vi "Ballast.vi"(11 "Full System Configuration":T1={"Rack"=enum."15U; 1-Phase; 16A; 100-240V", "Middle Rail"=enum."None", "Ballast"={"Main"=0, "Small"=0, "Side"=0}, "Front Panel I/O"={"EMO Button"=FALSE, "USB 3.0"=FALSE, "Display"=FALSE, "1st USB 2.0"=FALSE, "2nd USB 2.0"=FALSE, "Ethernet 3"=FALSE, "EMO Extension (3rd Party)"=FALSE, "EMO Extension (Rack In & Out)"=FALSE, "Aux Dual C13 QAC Outlets"=FALSE, "Residual-current Circuit Breaker"=FALSE, "Serial"=FALSE, "GPIB"=FALSE}, "Rear Panel I/O"={"Rear Panel I/O Configuration"=enum."Blank Panel", "EMO Button"=FALSE, "Power, Status & Banana Ground"=FALSE, "Ethernet 2"=FALSE, "Display"=FALSE, "USB 3.0"=FALSE, "DIO"=FALSE, "GPIB"=FALSE, "Aux Dual C13 QAC Outlets"=FALSE, "Residual-current Circuit Breaker"=FALSE, "Serial"=FALSE, "SMA"=FALSE}, "Miscellaneous Options"={"Eyebolts"=FALSE, "Tower Light"=FALSE, "Top/Side Monitor Mount Kit"=FALSE, "24\" Monitor"=FALSE, "Keyboard & Mouse"=FALSE, "Secondary Ethernet Switch"=FALSE, "Extra USB Hub"=FALSE, "USB-6509"=FALSE, "Front Door"=enum."38U (Solid) IG", "Primary Ethernet Switch"=enum."Item 0", "Use Posture"=enum."Item 0"}, "Accessories"={"Screw Type"=enum."10-32", "Cage Nuts & Screws"=0.0, "Filler Panel Color"=enum."Interface Gray", "1U"=0.0, "2U"=0.0, "3U"=0.0}} {"Ballast"."Side" max=5 step=1; "Ballast"."Small" max=5 step=1; "Ballast"."Main" max=5 step=1}) -> (3 "Array":T13[](array[typedef]))   [LabVIEW 2023]
uses:
  Option Type Defs/Parts List.ctl
  Option Type Defs/Full System Configuration.ctl
  Option Type Defs/Rack.ctl
  Option Type Defs/Middle Rail.ctl
  Option Type Defs/Ballast.ctl
  Option Type Defs/Front Panel IO.ctl
  Option Type Defs/Rear Panel IO.ctl
  Option Type Defs/Rear Panel IO Configuration.ctl
  Option Type Defs/Miscellaneous Options.ctl
  Option Type Defs/Front Door.ctl
  Option Type Defs/Accessories.ctl
  Option Type Defs/Screw Types.ctl
  Option Type Defs/Filler Panel Color.ctl
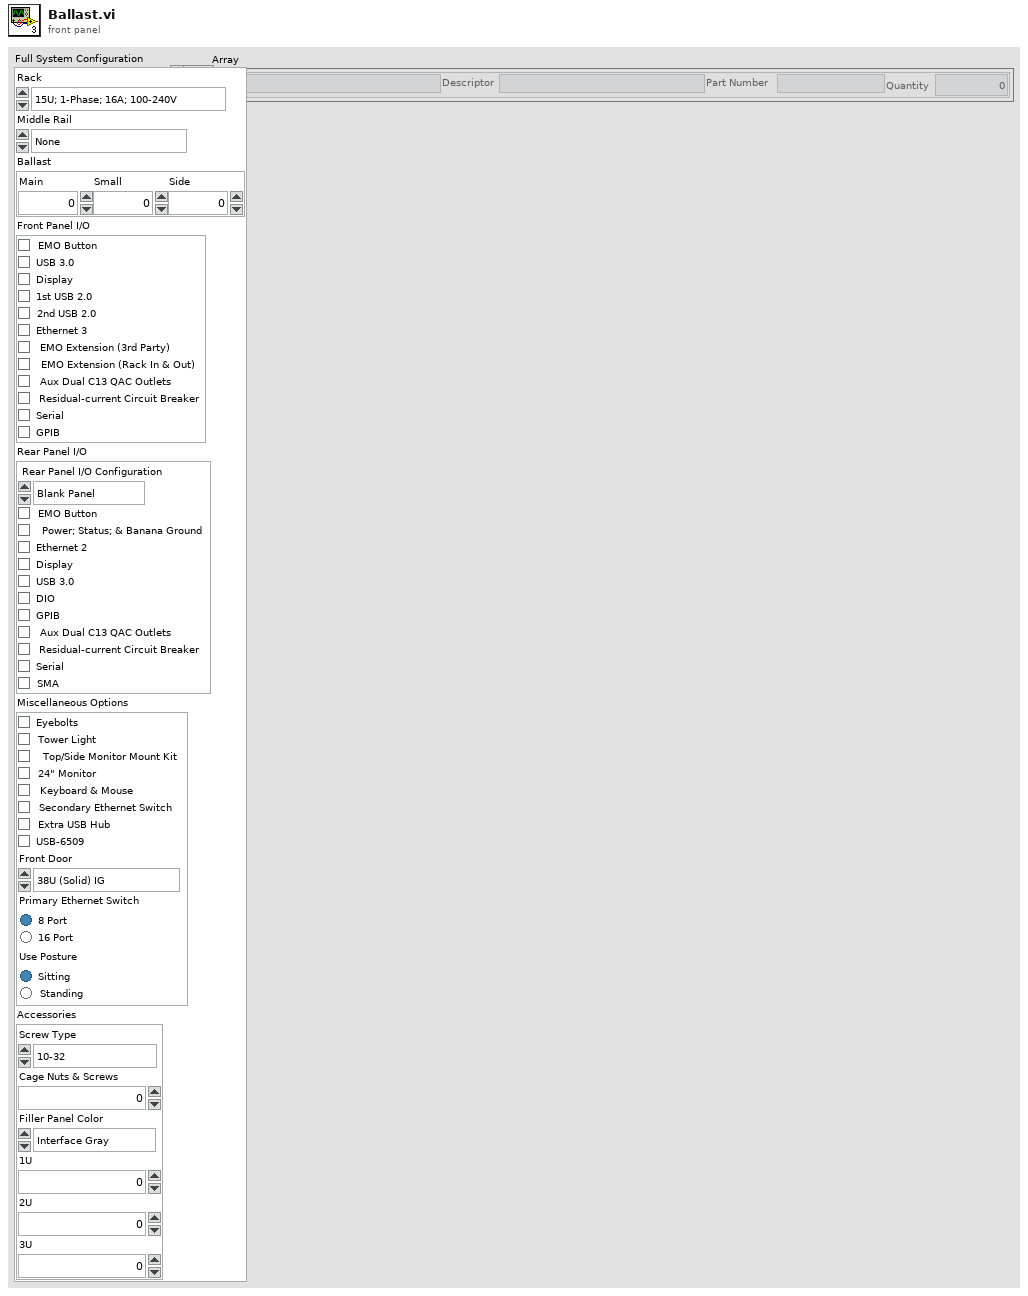
[diagram p1: front panel]
types:
  T1 = typedef "Full System Configuration.ctl" = cluster{"Rack":T2, "Middle Rail":T3, "Ballast":T4, "Front Panel I/O":T5, "Rear Panel I/O":T6, "Miscellaneous Options":T8, "Accessories":T10}
  T2 = typedef "Rack.ctl" = enum16{"15U; 1-Phase; 16A; 100-240V", "15U; 1-Phase; 24A; 100-240V", "38U; 3-Phase Delta; 50A; 200-240V", "38U; 1-Phase; 24A; 100-120V", "38U; 3-Phase Wye; 50A; 200-240V", "38U; 3-Phase Delta; 50A; 380-480V", "38U; 3-Phase Delta; 32A; 200-240V", "38U; 3-Phase Wye; 16A; 100-240V", "44U; 1-Phase; 24A; 100-240V", "44U; 3-Phase Delta; 32A; 200-240V"}
  T3 = typedef "Middle Rail.ctl" = enum16{"None", "Flip Side Rear; D=168.83mm", "Parallel Rear; D=145mm", "Flip Side Front; D=145mm", "Parallel Front; D=145mm"}
  T4 = typedef "Ballast.ctl" = cluster{"Main":u16, "Small":u16, "Side":u16}
  T5 = typedef "Front Panel IO.ctl" = cluster{"EMO Button":bool, "USB 3.0":bool, "Display":bool, "1st USB 2.0":bool, "2nd USB 2.0":bool, "Ethernet 3":bool, "EMO Extension (3rd Party)":bool, "EMO Extension (Rack In & Out)":bool, "Aux Dual C13 QAC Outlets":bool, "Residual-current Circuit Breaker":bool, "Serial":bool, "GPIB":bool}
  T6 = typedef "Rear Panel IO.ctl" = cluster{"Rear Panel I/O Configuration":T7, "EMO Button":bool, "Power, Status & Banana Ground":bool, "Ethernet 2":bool, "Display":bool, "USB 3.0":bool, "DIO":bool, "GPIB":bool, "Aux Dual C13 QAC Outlets":bool, "Residual-current Circuit Breaker":bool, "Serial":bool, "SMA":bool}
  T7 = typedef "Rear Panel IO Configuration.ctl" = enum16{"Blank Panel", "Fully Populated Panel", "Custom Panel"}
  T8 = typedef "Miscellaneous Options.ctl" = cluster{"Eyebolts":bool, "Tower Light":bool, "Top/Side Monitor Mount Kit":bool, "24\" Monitor":bool, "Keyboard & Mouse":bool, "Secondary Ethernet Switch":bool, "Extra USB Hub":bool, "USB-6509":bool, "Front Door":T9, "Primary Ethernet Switch":enum32{"Item 0", "Item 1"}, "Use Posture":enum32{"Item 0", "Item 1"}}
  T9 = typedef "Front Door.ctl" = enum16{"None", "38U (Solid) IG", "38U (Solid) EG", "38U: Top 14U (Solid) IG", "38U (Clear) IG", "44U (Solid) IG", "44U (Solid) EG"}
  T10 = typedef "Accessories.ctl" = cluster{"Screw Type":T11, "Cage Nuts & Screws":dbl, "Filler Panel Color":T12, "1U":dbl, "2U":dbl, "3U":dbl}
  T11 = typedef "Screw Types.ctl" = enum16{"None", "M6 (Most Common)", "10-32", "12-24"}
  T12 = typedef "Filler Panel Color.ctl" = enum16{"None", "Interface Gray", "Environmental Gray"}
  T13 = typedef "Parts List.ctl" = cluster{"Part":string, "Descriptor":string, "Part Number":string, "Quantity":dbl}
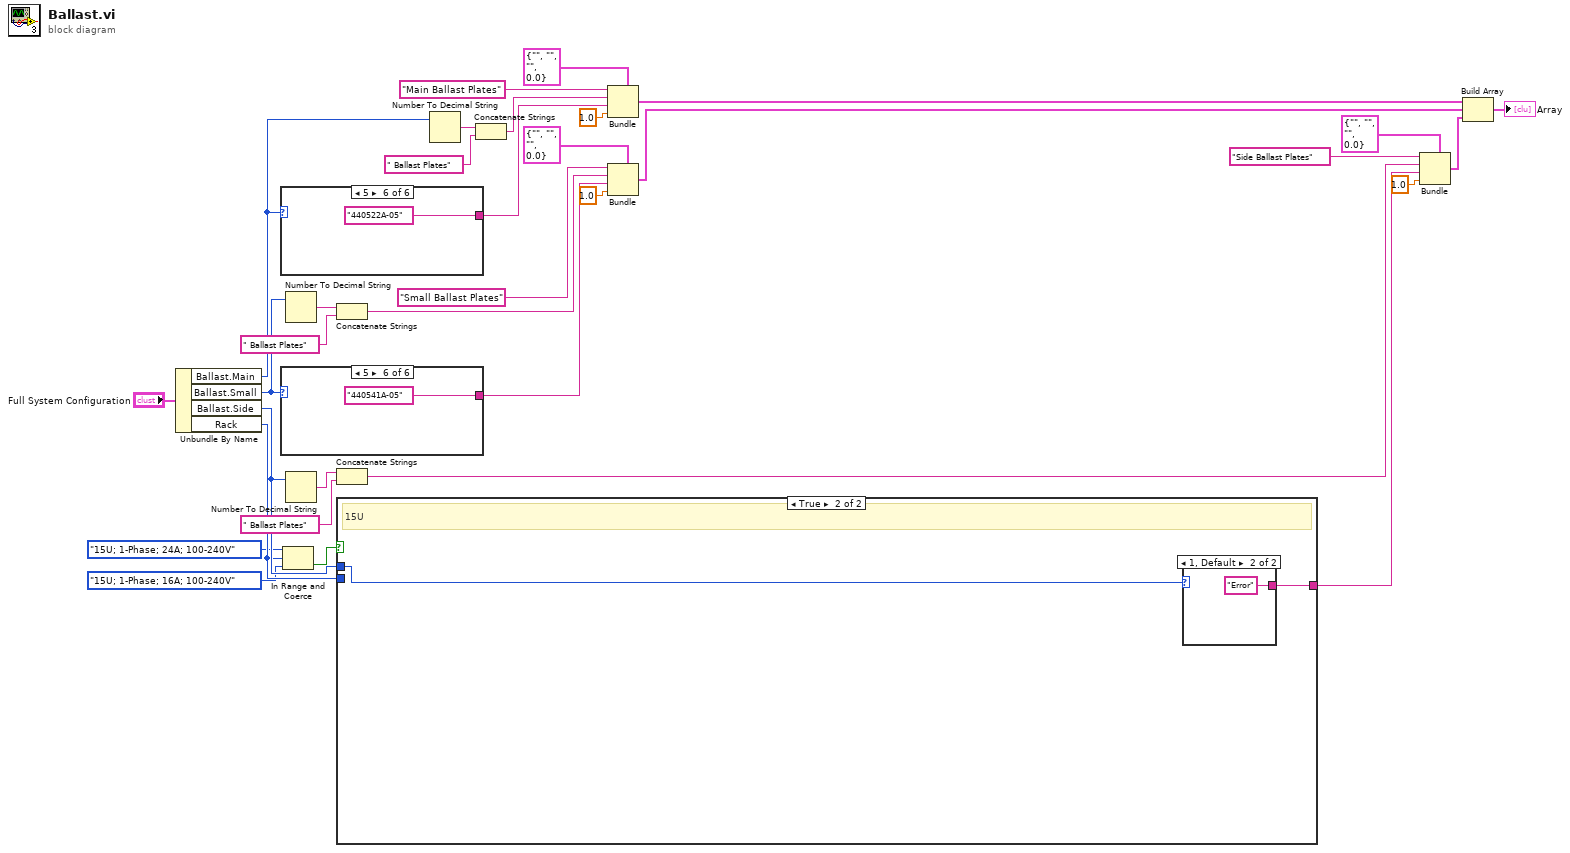
[diagram p0: block diagram]
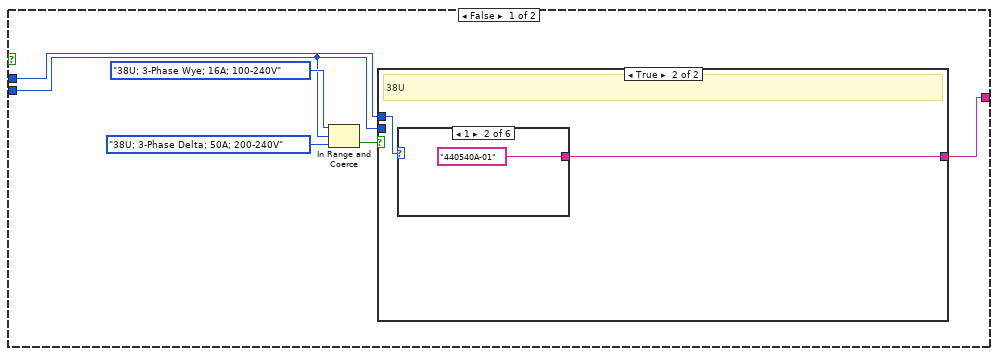
[diagram p2: hidden frame]
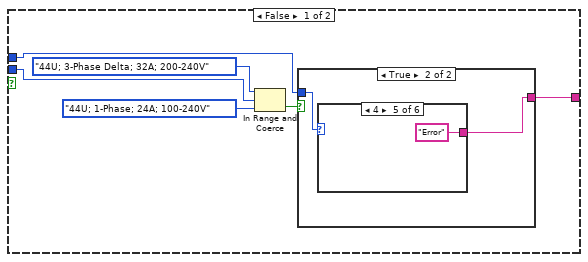
[diagram p3: hidden frame]
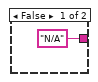
[diagram p4: hidden frame]
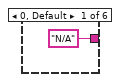
[diagram p5: hidden frame]
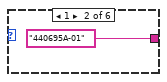
[diagram p6: hidden frame]
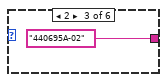
[diagram p7: hidden frame]
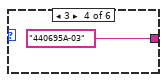
[diagram p8: hidden frame]
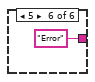
[diagram p9: hidden frame]
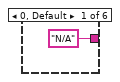
[diagram p10: hidden frame]
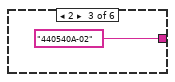
[diagram p11: hidden frame]
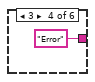
[diagram p12: hidden frame]
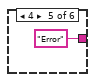
[diagram p13: hidden frame]
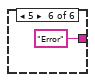
[diagram p14: hidden frame]
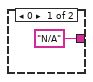
[diagram p15: hidden frame]
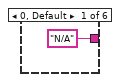
[diagram p16: hidden frame]
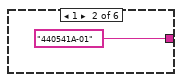
[diagram p17: hidden frame]
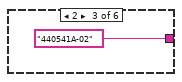
[diagram p18: hidden frame]
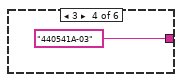
[diagram p19: hidden frame]
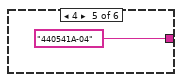
[diagram p20: hidden frame]
diagram:
  n1 = Unbundle By Name("Full System Configuration") -> ("Ballast.Main"=w28:u16, "Ballast.Small"=w30:u16, "Ballast.Side"=w33:u16, "Rack"=w17:T2)
  n2 = case shown="5" w28 {
    tunnel: ["N/A" "440522A-01" "440522A-02" "440522A-03" "440522A-04" "440522A-05"] -> w21
    frame 0, Default {
    }
    frame 1 {
    }
    frame 2 {
    }
    frame 3 {
    }
    frame 4 {
    }
    frame 5 {
    }
  }
  n3 = case shown="5" w30 {
    tunnel: ["N/A" "440541A-01" "440541A-02" "440541A-03" "440541A-04" "440541A-05"] -> w23
    frame 0, Default {
    }
    frame 1 {
    }
    frame 2 {
    }
    frame 3 {
    }
    frame 4 {
    }
    frame 5 {
    }
  }
  n4 = In Range and Coerce(upper limit=Rack."15U; 1-Phase; 24A; 100-240V" ("Rack"), x=w17, lower limit=Rack."15U; 1-Phase; 16A; 100-240V" ("Rack")) -> (In Range?=w16:bool)  [unwired: 1 out]
  n5 = Number To Decimal String(number=w30) -> (decimal integer string=w8:string)  [unwired: 1 in]
  n6 = Number To Decimal String(number=w33) -> (decimal integer string=w2:string)  [unwired: 1 in]
  n7 = Concatenate Strings(w8, " Ballast Plates" ("string")) -> (w7:string)
  n8 = Concatenate Strings(w2, " Ballast Plates" ("string")) -> (w1:string)
  n9 = case shown="True" w16 {
    tunnel: [w51 w76] -> w24
    tunnel: w17 -> [w47 _]
    tunnel: w33 -> [w46 w75]
    frame False {
      n10 = In Range and Coerce(upper limit=Rack."38U; 3-Phase Wye; 16A; 100-240V" ("Rack"), x=w47, lower limit=Rack."38U; 3-Phase Delta; 50A; 200-240V" ("Rack")) -> (In Range?=w48:bool)  [unwired: 1 out]
      n11 = case shown="True" w48 {
        tunnel: [w53 w68] -> w51
        tunnel: w47 -> [w55 _]
        tunnel: w46 -> [w52 w67]
        frame False {
          n12 = In Range and Coerce(upper limit=Rack."44U; 3-Phase Delta; 32A; 200-240V" ("Rack"), x=w55, lower limit=Rack."44U; 1-Phase; 24A; 100-240V" ("Rack")) -> (In Range?=w54:bool)  [unwired: 1 out]
          n13 = case shown="True" w54 {
            tunnel: ["N/A" w60] -> w53
            tunnel: w52 -> [_ w59]
            frame False {
            }
            frame True {
              n14 = case shown="4" w59 {
                tunnel: ["N/A" "440695A-01" "440695A-02" "440695A-03" "Error" "Error"] -> w60
                frame 0, Default {
                }
                frame 1 {
                }
                frame 2 {
                }
                frame 3 {
                }
                frame 4 {
                }
                frame 5 {
                }
              }
            }
          }
        }
        frame True {
          # "38U"
          n15 = case shown="1" w67 {
            tunnel: ["N/A" "440540A-01" "440540A-02" "Error" "Error" "Error"] -> w68
            frame 0, Default {
            }
            frame 1 {
            }
            frame 2 {
            }
            frame 3 {
            }
            frame 4 {
            }
            frame 5 {
            }
          }
        }
      }
    }
    frame True {
      # "15U"
      n16 = case shown="1, Default" w75 {
        tunnel: ["N/A" "Error"] -> w76
        frame 0 {
        }
        frame 1, Default {
        }
      }
    }
  }
  n17 = Number To Decimal String(number=w28) -> (decimal integer string=w4:string)  [unwired: 1 in]
  n18 = Concatenate Strings(w4, " Ballast Plates" ("string")) -> (w3:string)
  n19 = Bundle(cluster=T13 {"Part"="", "Descriptor"="", "Part Number"="", "Quantity"=0.0}, "Part"="Main Ballast Plates", "Descriptor"=w3, "Part Number"=w21, "Quantity"=1.0) -> (w22:T13)
  n20 = Bundle(cluster=T13 {"Part"="", "Descriptor"="", "Part Number"="", "Quantity"=0.0}, "Part"="Small Ballast Plates", "Descriptor"=w7, "Part Number"=w23, "Quantity"=1.0) -> (w25:T13)
  n21 = Bundle(cluster=T13 {"Part"="", "Descriptor"="", "Part Number"="", "Quantity"=0.0}, "Part"="Side Ballast Plates", "Descriptor"=w1, "Part Number"=w24, "Quantity"=1.0) -> (w26:T13)
  n22 = Build Array(w22, w25, w26) -> (→"Array":T13[])
